vi "Config Brightness.vi"(0 "VISA resource name":refnum<visa-resource-name>, 5 "Capacitance (5)":i32=5 max=9, 7 "Loss (5)":u16=5 max=9, 9 "Others (5)":u16=5 max=9, 11 "error in":errorcluster) -> (4 "VISA resource name out":refnum<visa-resource-name>, 15 "error out":errorcluster)   [LabVIEW 2019, in "Andeen-Hagerling 2700(400 firmware).lvlib"]
doc: "Sets the brightness of the front panel capacitance display, loss display and the frequency display and status and units and indicators."
uses:
  Andeen-Hagerling 2700(400 firmware).lvlib
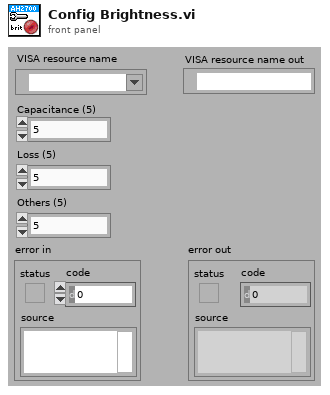
[diagram p1: front panel]
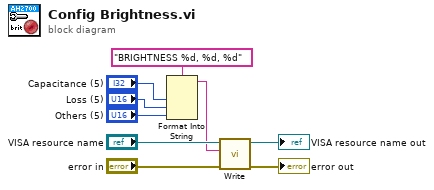
[diagram p0: block diagram]
diagram:
  n1 = Format Into String(format string="BRIGHTNESS %d, %d, %d", "Capacitance (5)", "Loss (5)", "Others (5)") -> (resulting string=w1:string)  [unwired: 2 in, 1 out]
  n2 = call "Write.vi"("error in"="error in", "command"=w1, "VISA resource name"="VISA resource name") -> ("error out"=→"error out":errorcluster, "VISA resource name out"=→"VISA resource name out":refnum<visa-resource-name>)  [unwired: 7 in]
